vi "Read Event Data.vi"(11 "Event Generated Msg":refnum<class "Event Generated Msg.lvclass">) -> (2 "Event Data":refnum<class "Event.lvclass">)   [LabVIEW 2015, in "Event Source.lvlib" / "Event Generated Msg.lvclass"]
doc: "Read the event data from the abstract Event Generated Msg sent to registrant. This method should be called within the registrants Do.vi specified to handle Event Generated Msg abstract message."
uses:
  Event Generated Msg.lvclass
  Event/Event.lvclass
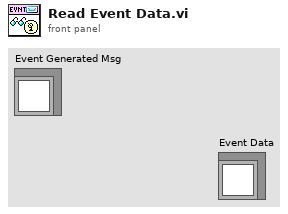
[diagram p1: front panel]
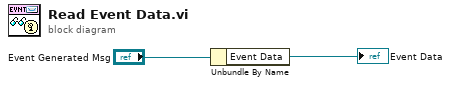
[diagram p0: block diagram]
diagram:
  n1 = Unbundle By Name ("Attribute Unbundler")("Event Generated Msg") -> ("Event Data"=→"Event Data":refnum<class "Event.lvclass">)
